vi "merge_labels_and_value_pairs.vi"(9 "Format string":string, 10 "Value Pairs":T2={"Data Array"=[], "Show ticks"=TRUE, "Show grid lines"=TRUE, "Labels"=enum."Value"}, 11 "Data Array":sgl[](array[numeric])) -> (2 "Merged Array Out":T1(array[cluster]))   [LabVIEW 2020, in "3DPC_SurfacePlot.xctl"]
uses:
  <vilib>/Native 3D Graph/xcontrol/3DPC_SurfacePlot.xctl
  <vilib>/Native 3D Graph/typedefs/prop_value_pair_1d.ctl
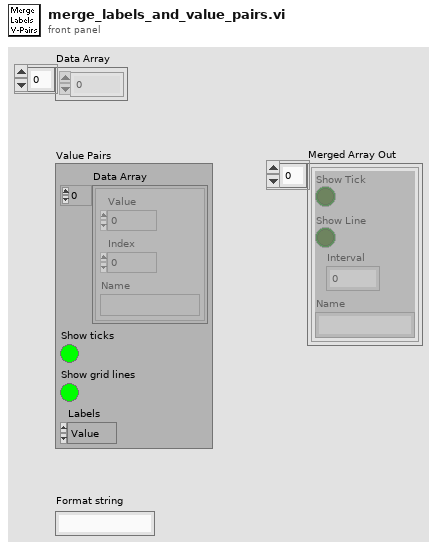
[diagram p1: front panel]
types:
  T1 = cluster{"Show Tick":bool, "Show Line":bool, "Interval":sgl, "Name":string}[]
  T2 = typedef "3DPC_SurfacePlot.xctl/prop_value_pair_1d.ctl" = cluster{"Data Array":cluster{"Value":sgl, "Index":i32, "Name":string}[], "Show ticks":bool, "Show grid lines":bool, "Labels":enum16{"Value", "None", "Name"}}
  T3 = cluster{"Show ticks":bool, "Show grid lines":bool, "Value":sgl, "Name":string}[]
  T4 = cluster{"Value":sgl, "Index":i32, "Name":string}[]
  T5 = cluster{"Show ticks":bool, "Show grid lines":bool, "Value":sgl, "Name":string}
  T6 = cluster{"Show ticks":bool, "Show ticks":bool, "Interval":sgl, string}
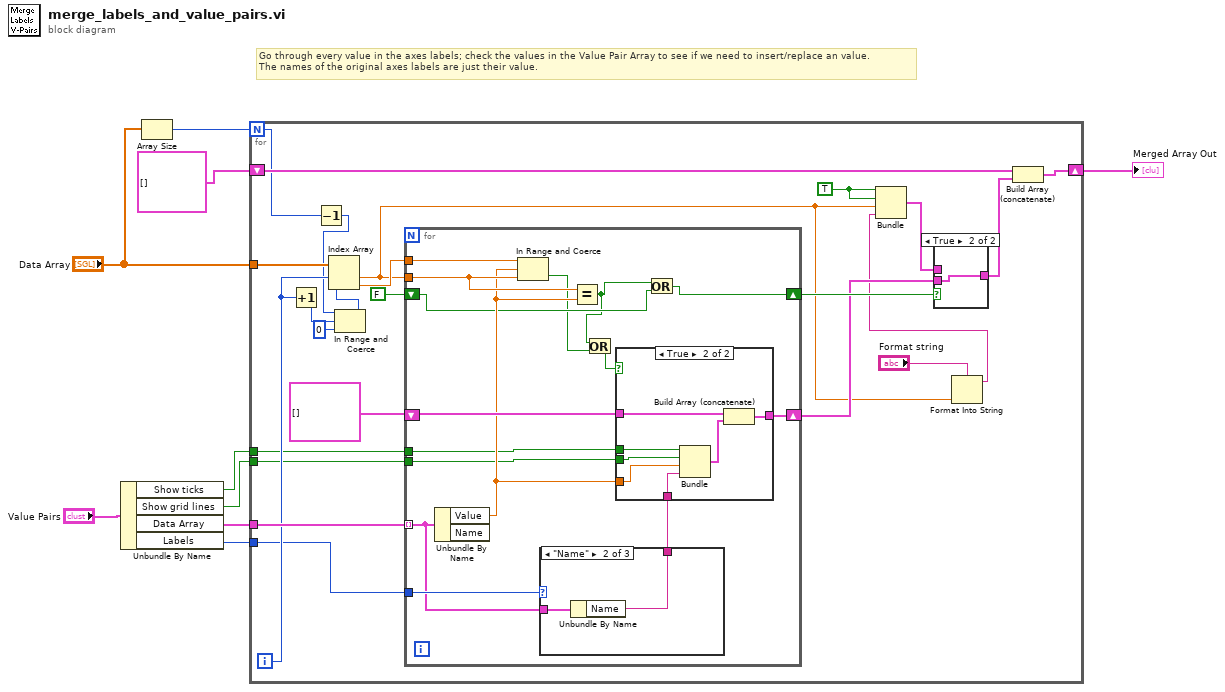
[diagram p0: block diagram]
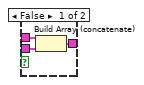
[diagram p2: hidden frame]
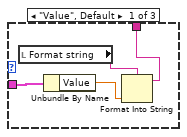
[diagram p3: hidden frame]
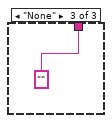
[diagram p4: hidden frame]
diagram:
  # "Go through every value in the axes labels; check the values in the Value Pair Array to see if we need to insert/replace an value.\nThe names of the original axes labels are just their value."
  n1 = Unbundle By Name("Value Pairs") -> ("Show ticks"=w5:bool, "Show grid lines"=w4:bool, "Data Array"=w8:T4, "Labels"=w7:enum16{"Value", "None", "Name"})
  n2 = Array Size(array="Data Array") -> (size(s)=w2:i32)
  n3 = for {
    N: w2 -> [w12]
    tunnel: "Data Array" -> [w32]
    tunnel: w8 -> [w33]
    tunnel: w7 -> [w30]
    shift-right: [w24] -> w1
    shift-left: T3 [] -> [w20]
    tunnel: w5 -> [w23]
    tunnel: w4 -> [w22]
    i -> [w31]
    w19 = TRUE ("Show ticks")
    n4 = Increment(x=w31) -> (x+1=w14:i32)
    n5 = Decrement(x=w12) -> (x-1=w11:i32)
    n6 = In Range and Coerce(upper limit=w11, x=w14, lower limit=0) -> (coerced(x)=w10:i32)  [unwired: 1 out]
    n7 = Index Array(array=w32, index #1=w31, index #2=w10) -> (element #1=w18:sgl, element #2=w29:sgl)
    n8 = for {
      tunnel: w33 -> [w47] mode=indexing
      tunnel: w29 -> [w52]
      tunnel: w18 -> [w51]
      tunnel: w30 -> [w50]
      shift-right: [w45] -> w26
      shift-left: T3 [] -> [w49]
      tunnel: w23 -> [w44]
      tunnel: w22 -> [w43]
      shift-right: [w42] -> w28
      shift-left: FALSE -> [w41]
      n9 = Unbundle By Name(w47) -> ("Value"=w48:sgl)  [unwired: 1 out]
      n10 = In Range and Coerce(upper limit=w52, x=w48, lower limit=w51) -> (In Range?=w39:bool)  [unwired: 1 out]
      n11 = case shown="\"Name\"" w50 {
        tunnel: w47 -> [w56 w58 _]
        tunnel: [w55 w57 "" ("Name")] -> w46
        frame "Value", Default {
          n12 = local read "Format string"() -> (w53:string)
          n13 = Unbundle By Name(w56) -> ("Value"=w54:sgl)
          n14 = Format Into String(format string=w53, w54) -> (resulting string=w55:string)  [unwired: 2 in, 1 out]
        }
        frame "Name" {
          n15 = Unbundle By Name(w58) -> ("Name"=w57:string)
        }
        frame "None" {
        }
      }
      n16 = Equal?(x=w51, y=w48) -> (x = y?=w40:bool)
      n17 = Or(x=w40, y=w39) -> (x .or. y?=w38:bool)
      n18 = case shown="True" w38 {
        tunnel: w49 -> [w60 w67]
        tunnel: w48 -> [_ w66]
        tunnel: w46 -> [_ w65]
        tunnel: [w60 w64] -> w45
        tunnel: w44 -> [_ w63]
        tunnel: w43 -> [_ w62]
        frame False {
        }
        frame True {
          n19 = Bundle("Show ticks"=w63, "Show grid lines"=w62, "Value"=w66, "Name"=w65) -> (w61:T5)  [unwired: 1 out]
          n20 = Build Array (concatenate)(w67, w61) -> (w64:T3)
        }
      }
      n21 = Or(x=w40, y=w41) -> (x .or. y?=w42:bool)
    }
    n22 = Format Into String(format string="Format string", w18) -> (resulting string=w17:string)  [unwired: 2 in, 1 out]
    n23 = Bundle("Show ticks"=w19, "Show ticks"=w19, "Interval"=w18, w17) -> (w27:T6)  [unwired: 1 out]
    n24 = case shown="True" w28 {
      tunnel: w27 -> [w36 _]
      tunnel: w26 -> [w35 w37]
      tunnel: [w34 w37] -> w25
      frame False {
        n25 = Build Array (concatenate)(w36, w35) -> (w34:T3)
      }
      frame True {
      }
    }
    n26 = Build Array (concatenate)(w20, w25) -> (w24:T3)
  }
  "Merged Array Out" <- w1
